vi "Init Histogram.vi"(8 "error in (no error)":errorcluster, 11 "Tosca in":refnum<class "Parameters.lvclass">) -> (0 "error out":errorcluster, 2 "Data":T1[](array[typedef]), 3 "Tosca out":refnum<class "Parameters.lvclass">)   [LabVIEW 2015, in "Parameters.lvclass"]
uses:
  Parameters.lvclass
  Histogram Data.ctl
  Parameters.lvclass/Parameters.ctl
  State/State.lvclass/State.ctl
  Timeout/Timeout.lvclass/Timeout.ctl
  Termination/Termination.lvclass/Termination.ctl
  Timeout/Write Result.vi
  Timeout/Read Result.vi
  Timeout/Read Color.vi
  Timeout/Read Type.vi
  Termination/Write Result.vi
  Termination/Read Result.vi
  Termination/Read Color.vi
  Termination/Read Type.vi
  State/Read Term.vi
  State/Read Timeouts.vi
  State/Write Term.vi
  State/Write Timeouts.vi
  Termination/Termination.lvclass
  Timeout/Timeout.lvclass
  State/State.lvclass
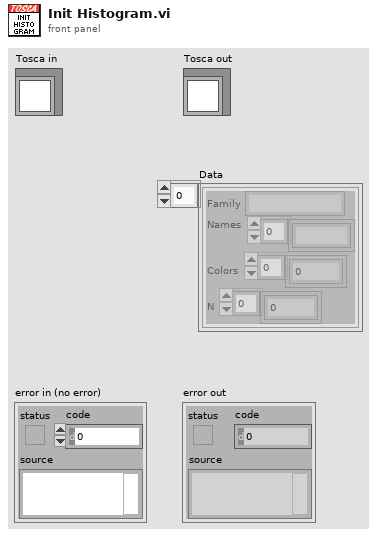
[diagram p1: front panel]
types:
  T1 = typedef "Parameters.lvclass/Histogram Data.ctl" = cluster{"Family":string, "Names":string[], "Colors":u32[], "N":i32[]}
  T2 = cluster{"Family":string, "Names":string[], "Colors":u32[], "N":i32[]}
  T3 = typedef "Tosca-Event Type.ctl" = enum16{"Normal", "CS+", "CS-"}
  T4 = typedef "Tosca-Parameter Family.ctl" = cluster{"Name":string, "Number":i32, "Vars":T5[], "Mask":bool[][], "one each":bool}
  T5 = typedef "Tosca-Parameter Table Element.ctl" = cluster{"state":string, "chan":string, "param":string, "expr":string, "dim":T6, "value":dbl[]}
  T6 = typedef "Tosca-Parameter Dimension.ctl" = enum16{"Ind", "X", "Y"}
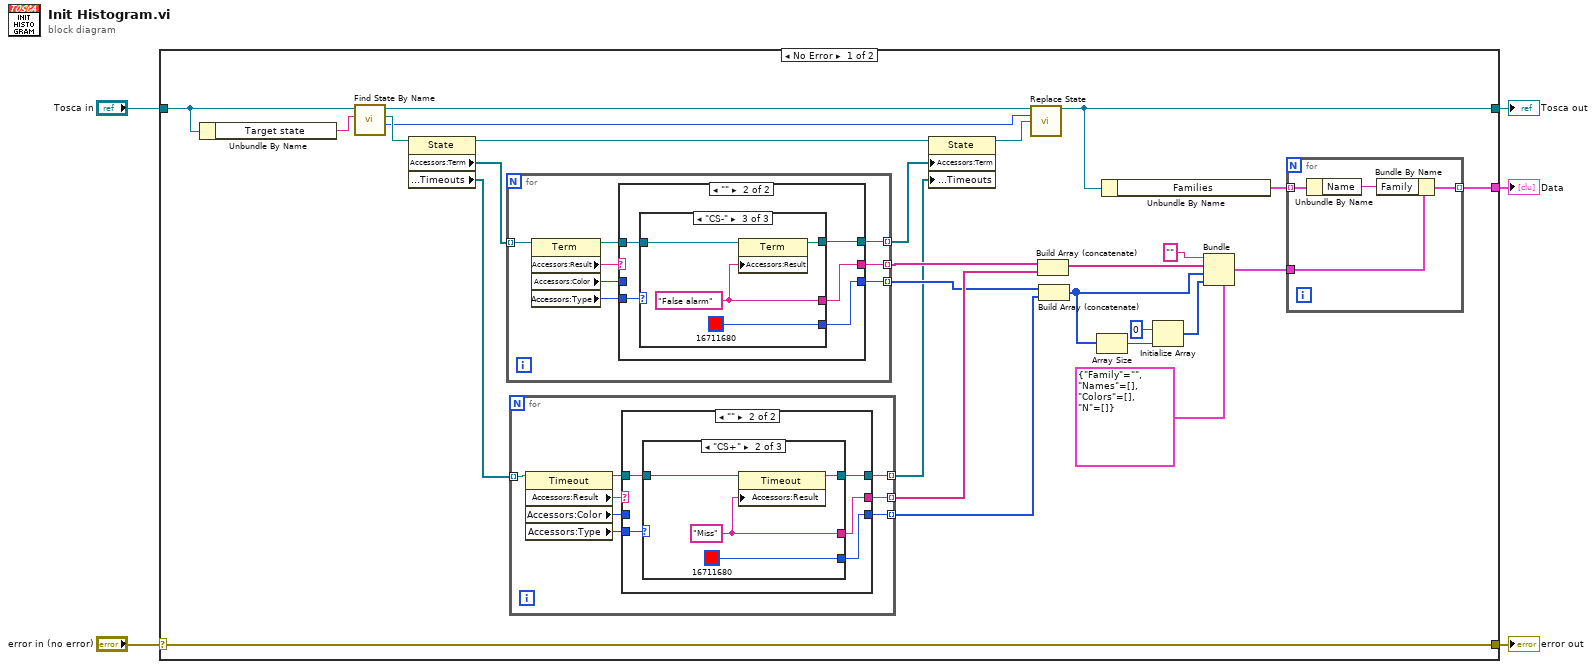
[diagram p0: block diagram]
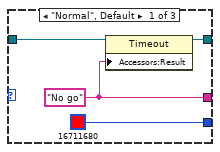
[diagram p3: hidden frame]
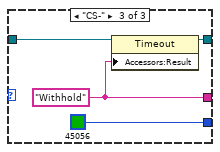
[diagram p4: hidden frame]
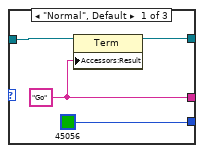
[diagram p6: hidden frame]
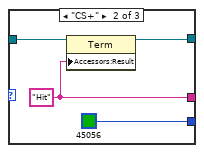
[diagram p7: hidden frame]
diagram:
  n1 = case shown="No Error" "error in (no error)" {
    selector: "error in (no error)" -> [w32 w94]
    tunnel: [w32 w94] -> w4
    tunnel: [w8 w93] -> w2
    tunnel: "Tosca in" -> [w28 w93]
    tunnel: [w13 _] -> w1
    frame No Error {
      n2 = Unbundle By Name(w28) -> ("Target state"=w31:string)
      n3 = call "Find State By Name.vi"("Name"=w31, "Tosca in"=w28) -> ("Index"=w7:i32, "State"=w30:refnum<class "State.lvclass">, "Tosca out"=w9:refnum<class "Parameters.lvclass">)  [unwired: 6 in, 1 out]
      n4 = property class="State"(reference=w30) -> (reference out=w12:refnum<class "State.lvclass">, "Accessors:Term"=w29:refnum<class "Termination.lvclass">[], "Accessors:Timeouts"=w27:refnum<class "Timeout.lvclass">[])  [unwired: 1 in, 1 out]
      n5 = for {
        tunnel: w29 -> [w72] mode=indexing
        tunnel: [w69] -> w26 mode=indexing
        tunnel: [w67] -> w24 mode=indexing
        tunnel: [w65] -> w11 mode=indexing
        n6 = property class="Term"(reference=w72) -> (reference out=w66:refnum<class "Termination.lvclass">, "Accessors:Result"=w71:string, "Accessors:Color"=w68:u32, "Accessors:Type"=w70:T3)  [unwired: 1 in, 1 out]
        n7 = case shown="\"\"" w71 {
          selector: w71 -> [w75 _]
          tunnel: [w75 w79] -> w69
          tunnel: w70 -> [_ w80]
          tunnel: w68 -> [w74 _]
          tunnel: [w74 w78] -> w67
          tunnel: w66 -> [w73 w77]
          tunnel: [w73 w76] -> w65
          frame "something", Default {
          }
          frame "" {
            n8 = case shown="\"CS-\"" w80 {
              tunnel: [w82 w85 w89] -> w79
              tunnel: [u32 45056 u32 45056 u32 16711680] -> w78
              tunnel: w77 -> [w83 w87 w91]
              tunnel: [w81 w86 w90] -> w76
              frame "Normal", Default {
                w82 = "Go"
                n9 = property class="Term"(reference=w83, "Accessors:Result"=w82) -> (reference out=w81:refnum<class "Termination.lvclass">)  [unwired: 1 in, 1 out]
              }
              frame "CS+" {
                w85 = "Hit"
                n10 = property class="Term"(reference=w87, "Accessors:Result"=w85) -> (reference out=w86:refnum<class "Termination.lvclass">)  [unwired: 1 in, 1 out]
              }
              frame "CS-" {
                w89 = "False alarm"
                n11 = property class="Term"(reference=w91, "Accessors:Result"=w89) -> (reference out=w90:refnum<class "Termination.lvclass">)  [unwired: 1 in, 1 out]
              }
            }
          }
        }
      }
      n12 = for {
        tunnel: w27 -> [w44] mode=indexing
        tunnel: [w41] -> w25 mode=indexing
        tunnel: [w39] -> w23 mode=indexing
        tunnel: [w37] -> w10 mode=indexing
        n13 = property class="Timeout"(reference=w44) -> (reference out=w38:refnum<class "Timeout.lvclass">, "Accessors:Result"=w43:string, "Accessors:Color"=w40:u32, "Accessors:Type"=w42:T3)  [unwired: 1 in, 1 out]
        n14 = case shown="\"\"" w43 {
          selector: w43 -> [w47 _]
          tunnel: [w47 w51] -> w41
          tunnel: w42 -> [_ w52]
          tunnel: w40 -> [w46 _]
          tunnel: [w46 w50] -> w39
          tunnel: w38 -> [w45 w49]
          tunnel: [w45 w48] -> w37
          frame "something", Default {
          }
          frame "" {
            n15 = case shown="\"CS+\"" w52 {
              tunnel: [w53 w57 w61] -> w51
              tunnel: [u32 16711680 u32 16711680 u32 45056] -> w50
              tunnel: w49 -> [w55 w58 w63]
              tunnel: [w54 w59 w62] -> w48
              frame "Normal", Default {
                w53 = "No go"
                n16 = property class="Timeout"(reference=w55, "Accessors:Result"=w53) -> (reference out=w54:refnum<class "Timeout.lvclass">)  [unwired: 1 in, 1 out]
              }
              frame "CS+" {
                w57 = "Miss"
                n17 = property class="Timeout"(reference=w58, "Accessors:Result"=w57) -> (reference out=w59:refnum<class "Timeout.lvclass">)  [unwired: 1 in, 1 out]
              }
              frame "CS-" {
                w61 = "Withhold"
                n18 = property class="Timeout"(reference=w63, "Accessors:Result"=w61) -> (reference out=w62:refnum<class "Timeout.lvclass">)  [unwired: 1 in, 1 out]
              }
            }
          }
        }
      }
      n19 = property class="State"(reference=w12, "Accessors:Term"=w11, "Accessors:Timeouts"=w10) -> (reference out=w6:refnum<class "State.lvclass">)  [unwired: 1 in, 1 out]
      n20 = call "Replace State.vi"("Tosca in"=w9, "stateIndex"=w7, "State"=w6) -> ("Tosca out"=w8:refnum<class "Parameters.lvclass">)  [unwired: 12 in]
      n21 = Build Array (concatenate)(w26, w25) -> (w20:string[])
      n22 = Build Array (concatenate)(w24, w23) -> (w19:u32[])
      n23 = Array Size(array=w19) -> (size(s)=w21:i32)
      n24 = Unbundle By Name(w8) -> ("Families"=w17:T4[])
      n25 = Initialize Array(0, w21) -> (w18:i32[])
      n26 = Bundle(cluster=T2 {"Family"="", "Names"=[], "Colors"=[], "N"=[]} ("output cluster"), "Family"="", "Names"=w20, "Colors"=w19, "N"=w18) -> (w16:T2)
      n27 = for {
        tunnel: w17 -> [w36] mode=indexing
        tunnel: w16 -> [w35]
        tunnel: [w33] -> w13 mode=indexing
        n28 = Unbundle By Name(w36) -> ("Name"=w34:string)
        n29 = Bundle By Name(cluster=w35, "Family"=w34) -> (w33:T2)
      }
    }
    frame Error {
    }
  }
  "error out" <- w4
  "Tosca out" <- w2
  "Data" <- w1
